vi "Convert Settings to String.vi"(8 "error in (no error)":errorcluster, 11 "Settings in":T1={"Plug-in Version"="", "Step Values"=[], "Only Execute When Test Running"=TRUE, "Reset Sequence When Test Starts"=TRUE, "Number of Sequence Steps"=0, "Num of Analog Channels"=0, "Num of Digital Channels"=0, "Delay Before Starting Sequence"=0.0, "Default Analog Values"=[], "Default Digital Values"=[], "Max Iterations"=0, "Use last value when stopped"=FALSE, "Prioritize exact values"=FALSE, "Enable advanced step timing"=FALSE, "Enable step conditions"=FALSE, "Show confirmation dialogs"=FALSE, "Start condition"="", "Enable re-triggering"=FALSE, "Stop condition"=""}) -> (0 "error out":errorcluster, 3 "String out":string)   [LabVIEW 2024, in "Output Sequencer.lvlib" / "Output Sequencer.lvclass"]
uses:
  Output Sequencer.lvclass
  Settings UI/Types/Settings.ctl
  Settings UI/Types/Step Settings.ctl
  efaceabb-c9f2-4e33-a34b-72f25354c9b8.vi
  Globals/Global Strings.vi
  <vilib>/JDP Science/JSONtext/Variant to JSON Text.vi
  <vilib>/JDP Science/JSONtext/LVClass Serializer/JSONtext LVClass Serializer.lvclass
  Settings UI/Settings UI.lvclass
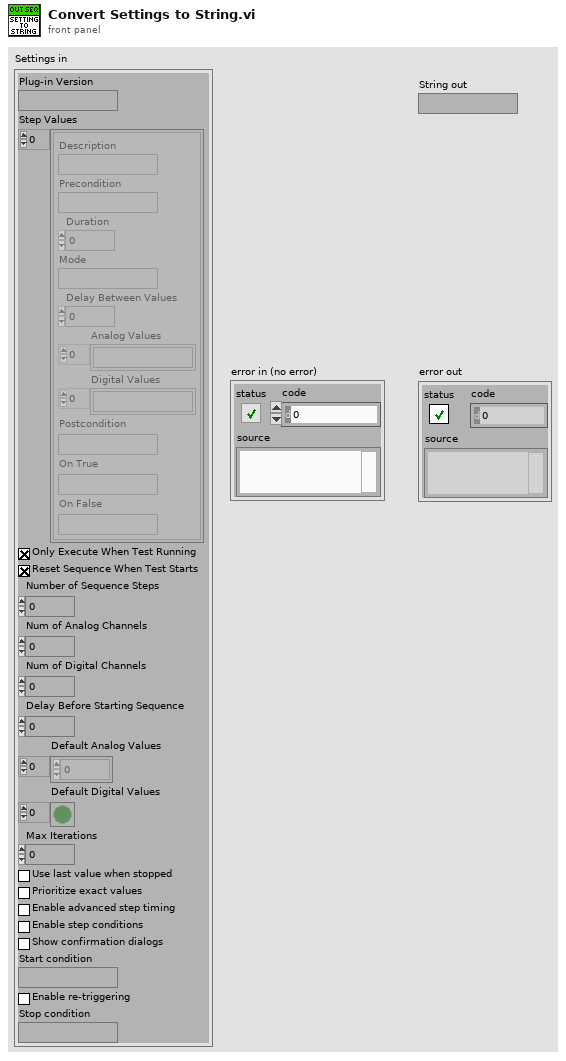
[diagram p1: front panel]
types:
  T1 = typedef "Output Sequencer.lvlib/Settings UI.lvclass/Settings.ctl" = cluster{"Plug-in Version":string, "Step Values":T2[], "Only Execute When Test Running":bool, "Reset Sequence When Test Starts":bool, "Number of Sequence Steps":i32, "Num of Analog Channels":i32, "Num of Digital Channels":i32, "Delay Before Starting Sequence":dbl, "Default Analog Values":dbl[], "Default Digital Values":bool[], "Max Iterations":u32, "Use last value when stopped":bool, "Prioritize exact values":bool, "Enable advanced step timing":bool, "Enable step conditions":bool, "Show confirmation dialogs":bool, "Start condition":string, "Enable re-triggering":bool, "Stop condition":string}
  T2 = typedef "Output Sequencer.lvlib/Settings UI.lvclass/Step Settings.ctl" = cluster{"Description":string, "Precondition":string, "Duration":dbl, "Mode":string, "Delay Between Values":dbl, "Analog Values":string[], "Digital Values":string[], "Postcondition":string, "On True":string, "On False":string}
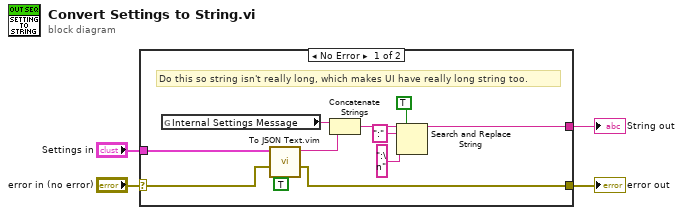
[diagram p0: block diagram]
diagram:
  n1 = case shown="No Error" "error in (no error)" {
    selector: "error in (no error)" -> [w5 w16]
    tunnel: [w15 _] -> w4
    tunnel: "Settings in" -> [w13 _]
    tunnel: [w6 w16] -> w2
    frame No Error {
      # "Do this so string isn't really long, which makes UI have really long string too."
      n2 = global read "Global Strings.vi" "Internal Settings Message"() -> (w14:string)
      n3 = call "To JSON Text.vim"("Pretty Print?"=TRUE, "error in (no error)"=w5, "Anything"=w13) -> ("error out"=w6:errorcluster, "<JSON>"=w8:string)  [unwired: 7 in]
      n4 = Concatenate Strings(w14, w8) -> (w12:string)
      n5 = Search and Replace String(replace all?=TRUE ("replace all? (F)"), input string=w12, search string=":", replace string=":\n" ("replace string (\"\")")) -> (result string=w15:string)  [unwired: 4 in, 3 out]
    }
    frame Error {
    }
  }
  "String out" <- w4
  "error out" <- w2
